vi "Anything to no Error Cluster.vi"(2 "Variant":variant) -> (7 "Error Out":errorcluster)   [LabVIEW 2021, in "Error.lvlib"]
uses:
  Error.lvlib
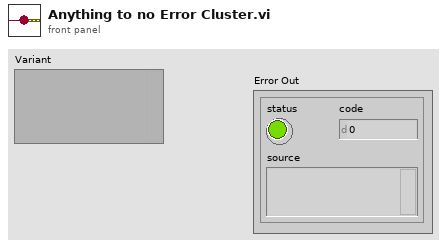
[diagram p1: front panel]
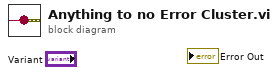
[diagram p0: block diagram]
diagram:
